vi "hSync&StartSampling2013.vi"(3 "error in":errorcluster, 4 "#Samples":u32=10000, 5 "FPGA VI Reference In":refnum<k20>) -> (0 "error out":errorcluster, 2 "FPGA VI Reference Out":refnum<k20>)   [LabVIEW 2014]
doc: "Gibt softwaregesteuert Sync-Impuls aus, Einlesende for-Schleife wird auf n Samples eingestellt und gestartet."
uses:
  <vilib>/Utility/error.llb/Error Cluster From Error Code.vi
  <vilib>/rvi/errors/niLvFpgaAdjustHostInterfaceError.vi
  <vilib>/rvi/interface/nirviReadWriteControl/nirviReadWriteControl.xnode
  FPGA Bitfiles/W7XBolo2017_FPGATarget_fmain2014_DACRangeVoltage.lvbitx
  f_main_2014.vi
  NiFpgaLv.dll
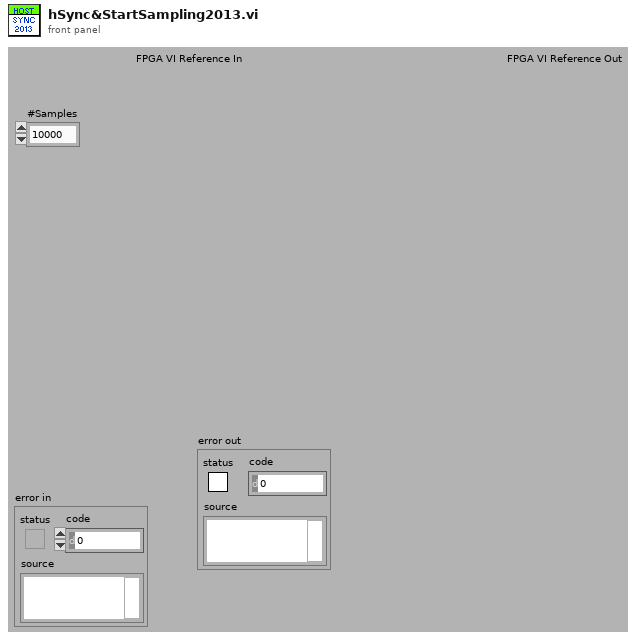
[diagram p1: front panel]
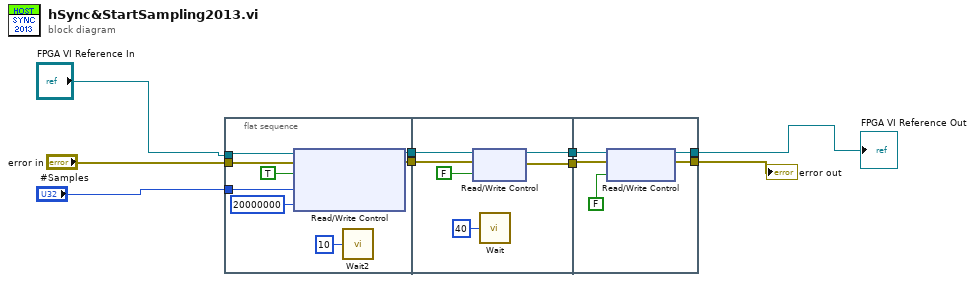
[diagram p0: block diagram]
diagram:
  n1 = flat-sequence {
    tunnel: [w16] -> w9
    tunnel: [w15] -> w8
    tunnel: "#Samples" -> [w14]
    tunnel: "FPGA VI Reference In" -> [w13]
    tunnel: "error in" -> [w12]
    tunnel: w9 -> [w20]
    tunnel: w8 -> [w19]
    tunnel: [w22] -> w5
    tunnel: [w21] -> w4
    tunnel: [w26] -> w2
    tunnel: w5 -> [w28]
    tunnel: w4 -> [w27]
    tunnel: [w25] -> w3
    frame #0 {
      n2 = xnode "Read/Write Control"("FPGA VI Reference In"=w13, "error in"=w12, "SYNC"=TRUE ("RESET"), "read_count"=w14, "Timeout(in Ticks)"=u32 20000000) -> ("FPGA VI Reference Out"=w16:refnum<k20>, "error out"=w15:errorcluster)
      n3 = call "Wait2"("Count(mSec)"=u32 10) -> ()  [unwired: 1 out]
    }
    frame #1 {
      n4 = xnode "Read/Write Control"("FPGA VI Reference In"=w20, "error in"=w19, "SYNC"=FALSE ("RESET")) -> ("FPGA VI Reference Out"=w22:refnum<k20>, "error out"=w21:errorcluster)
      n5 = call "Wait"("Count(mSec)"=u32 40) -> ()  [unwired: 1 out]
    }
    frame #2 {
      n6 = xnode "Read/Write Control"("FPGA VI Reference In"=w28, "error in"=w27, "ADCRead"=FALSE) -> ("FPGA VI Reference Out"=w26:refnum<k20>, "error out"=w25:errorcluster)
    }
  }
  "error out" <- w3
  "FPGA VI Reference Out" <- w2
